vi "Read_and_Write_Parameter_Test.vi"() -> ()   [LabVIEW 2017]
uses:
  Classes/ADCP.lvclass
  Classes/ADCP_Data_Packet_Transmit_Mode.ctl
panel:
  out "ADCP out":refnum<class "ADCP.lvclass">
  out "error out":errorcluster
  out "Data Packet out":T2
  out "Parameter Value Out":string
  in  "Parameter Value In":string
  in  "Parameter Name":string
  in  "Symbol File Path":path
  in  "error in (no error)":errorcluster
  in  "ADCP in":refnum<class "ADCP.lvclass">
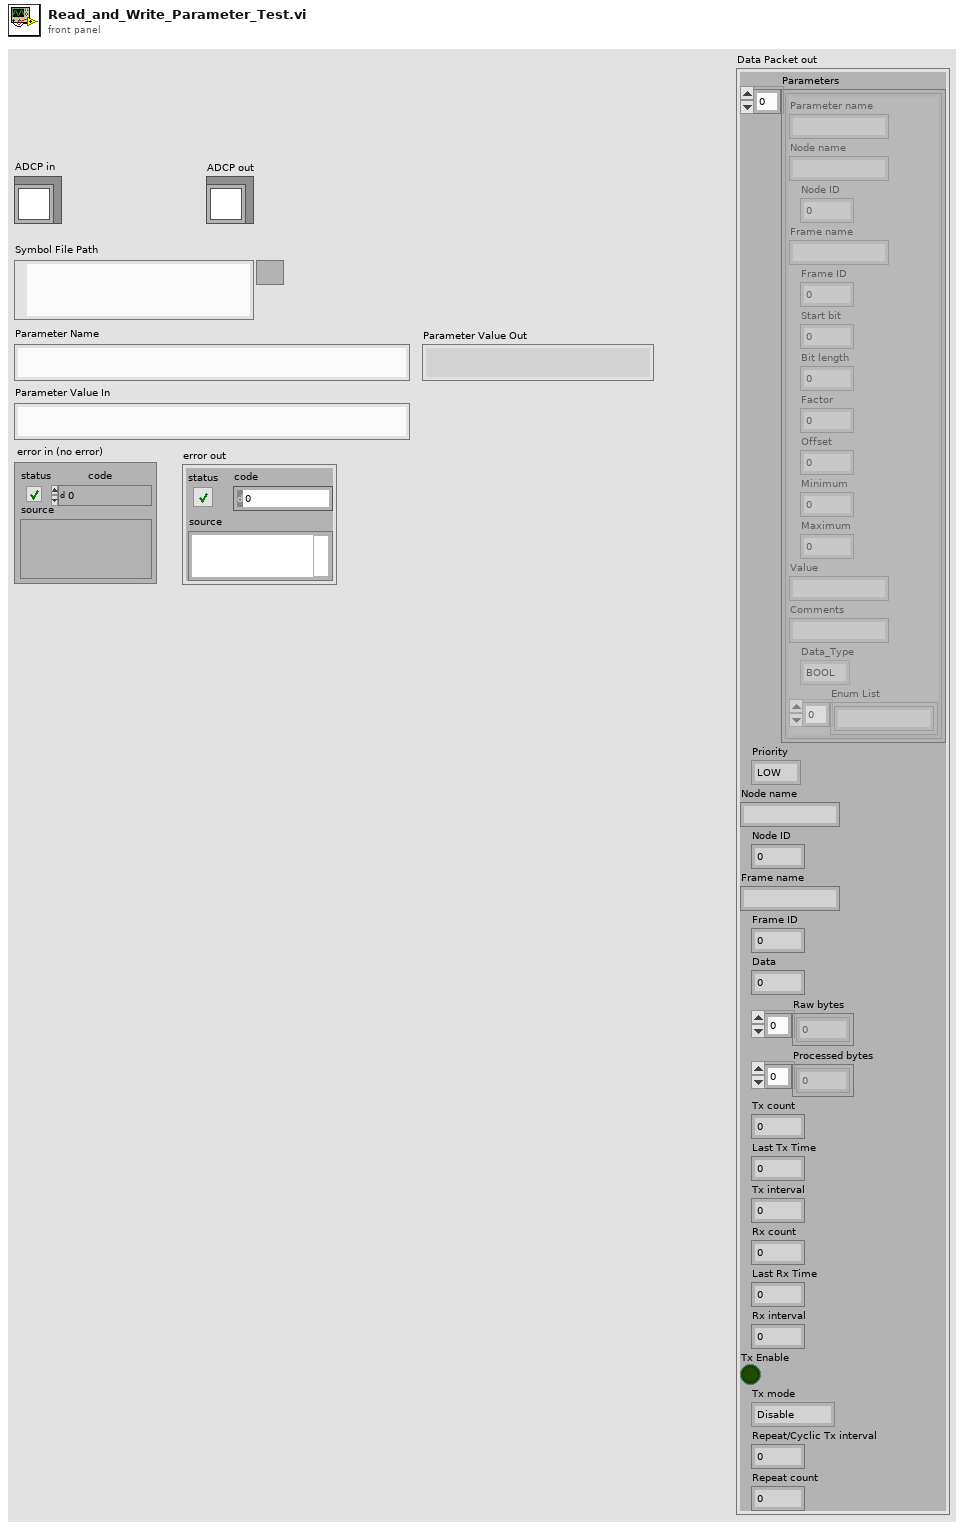
[diagram p1: front panel]
types:
  T1 = typedef "ADCP.lvclass/ADCP_Data_Packet_Transmit_Mode.ctl" = enum16{"Disable", "Single", "Cyclic", "Repeat"}
  T2 = cluster{"Parameters":cluster{"Parameter name":string, "Node name":string, "Node ID":u8, "Frame name":string, "Frame ID":u8, "Start bit":u32, "Bit length":u32, "Factor":dbl, "Offset":dbl, "Minimum":dbl, "Maximum":dbl, "Value":string, "Comments":string, "Data_Type":enum16{"BOOL", "UNSIGNED", "SIGNED", "FLOAT32", "ENUM"}, "Enum List":string[]}[], "Priority":enum16{"LOW", "HIGH"}, "Node name":string, "Node ID":u8, "Frame name":string, "Frame ID":u8, "Data":u32, "Raw bytes":u8[], "Processed bytes":u8[], "Tx count":i32, "Last Tx Time":u32, "Tx interval":u32, "Rx count":i32, "Last Rx Time":u32, "Rx interval":u32, "Tx Enable":bool, "Tx mode":T1, "Repeat/Cyclic Tx interval":u32, "Repeat count":u16}
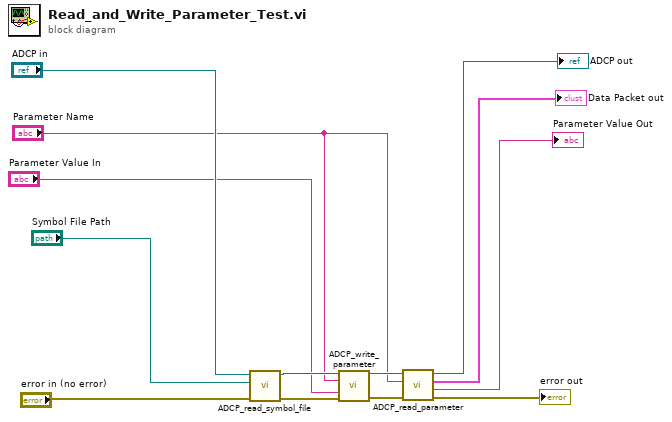
[diagram p0: block diagram]
diagram:
  n1 = call "ADCP_read_symbol_file.vi"("error in (no error)"="error in (no error)", "Symbol File Path"="Symbol File Path", "ADCP in"="ADCP in") -> ("error out"=w10:errorcluster, "ADCP out"=w9:refnum<class "ADCP.lvclass">)  [unwired: 5 in, 2 out]
  n2 = call "ADCP_write_parameter.vi"("ADCP in"=w9, "Parameter Name"="Parameter Name", "Parameter Value"="Parameter Value In", "error in (no error)"=w10) -> ("ADCP out"=w7:refnum<class "ADCP.lvclass">, "error out"=w6:errorcluster)  [unwired: 9 in, 1 out]
  n3 = call "ADCP_read_parameter.vi"("error in (no error)"=w6, "Parameter Name"="Parameter Name", "ADCP In"=w7) -> ("error out"=→"error out":errorcluster, "Parameter Value"=→"Parameter Value Out":string, "Data Packet out"=→"Data Packet out":T2, "ADCP out"=→"ADCP out":refnum<class "ADCP.lvclass">)  [unwired: 5 in]
